vi "Utility Maximum Flow.vi"(5 "Retry Attempts (0)":i32 min=0, 7 "Fast Comms (F)":bool, 8 "error in":errorcluster, 11 "VISA resource name":refnum<visa-resource-name>) -> (0 "error out":errorcluster, 2 "Maximum Flow":dbl, 3 "VISA resource name out":refnum<visa-resource-name>)   [LabVIEW 2020, in "ChromTech MX-Class Drivers.lvlib"]
doc: "Returns the maximum allowable flow rate for the pump in ml/min."
uses:
  <instrlib>/RxnRover/ChromtechNextGenDriver/ChromTech MX-Class Drivers.lvlib
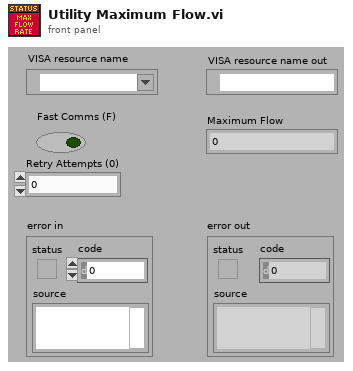
[diagram p1: front panel]
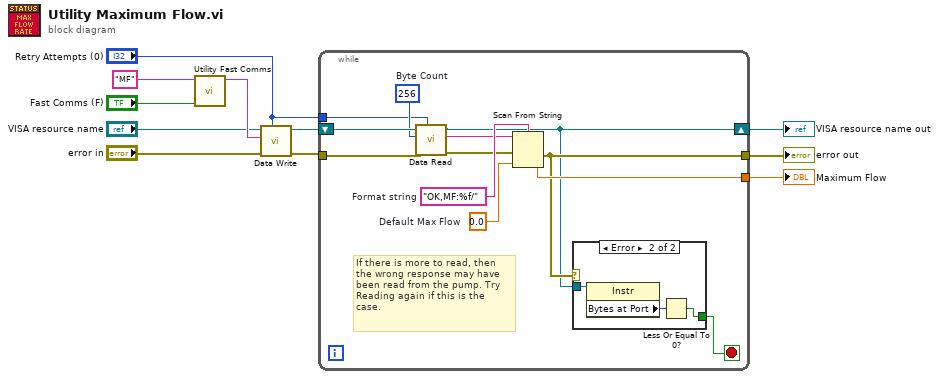
[diagram p0: block diagram]
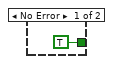
[diagram p2: hidden frame]
diagram:
  n1 = call <instrlib>:"Utility Fast Comms.vi"("Fast Comms"="Fast Comms (F)", "Command"="MF") -> ("Fast Command"=w8:string)  [unwired: 9 in]
  n2 = call <instrlib>:"Data Write.vi"("Retry Attempts (0)"="Retry Attempts (0)", "error in (no error)"="error in", "Command"=w8, "VISA Refnum in"="VISA resource name") -> ("error out"=w5:errorcluster, "VISA Refnum out"=w4:refnum<visa-resource-name>)  [unwired: 6 in]
  n3 = while {
    tunnel: [w22] -> w9
    tunnel: "Retry Attempts (0)" -> [w15]
    shift-right: [w13] -> w1
    shift-left: w4 -> [w17]
    tunnel: w5 -> [w18]
    tunnel: [w14] -> w2
    stop <- w12 stop-if-true
    w16 = 256  # Byte Count
    w21 = 0.0  # Default Max Flow
    w23 = "OK,MF:%f/"  # Format string
    # "If there is more to read, then\nthe wrong response may have\nbeen read from the pump. Try\nReading again if this is the\ncase."
    n4 = call <instrlib>:"Data Read.vi"("Retry Attempts (0)"=w15, "error in (no error)"=w18, "Bytes to read"=w16, "VISA Refnum in"=w17) -> ("error out"=w19:errorcluster, "read buffer"=w20:string, "VISA Refnum out"=w13:refnum<visa-resource-name>)  [unwired: 5 in]
    n5 = Scan From String(format string=w23, input string=w20, error in=w19, default 1=w21) -> (error out=w14:errorcluster, output 1=w22:dbl)  [unwired: 1 in, 2 out]
    n6 = case shown="Error" w14 {
      tunnel: w13 -> [_ w27]
      tunnel: [TRUE w25] -> w12
      frame No Error {
      }
      frame Error {
        n7 = property class="Instr"(reference=w27) -> ("Bytes at Port"=w26:u32)  [unwired: 1 in, 2 out]
        n8 = Less Or Equal To 0?(x=w26) -> (x <= 0?=w25:bool)
      }
    }
  }
  "VISA resource name out" <- w1
  "error out" <- w2
  "Maximum Flow" <- w9
